vi "Toggle.vi"(11 "booleanIn":bool) -> (3 "booleanOut":bool)   [LabVIEW 2018]
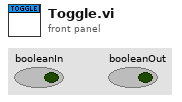
[diagram p1: front panel]
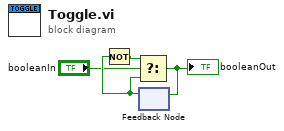
[diagram p0: block diagram]
diagram:
  n1 = feedback #1() -> (w2:bool)  [unwired: 1 in]
  n2 = Not(x=w2) -> (.not. x?=w3:bool)
  n3 = Select(t=w3, s="booleanIn", f=w2) -> (s? t:f=w4:bool)
  "booleanOut" <- w4
  n4 = feedback-in #1(w4) -> ()
